vi "add address to register list.vi"(0 "reference":refnum<vi>, 7 "RegisterAddress":i32, 13 "Register Selected":bool) -> ()   [LabVIEW 2010]
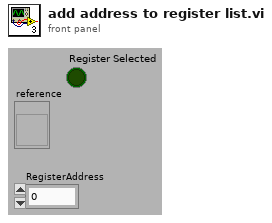
[diagram p1: front panel]
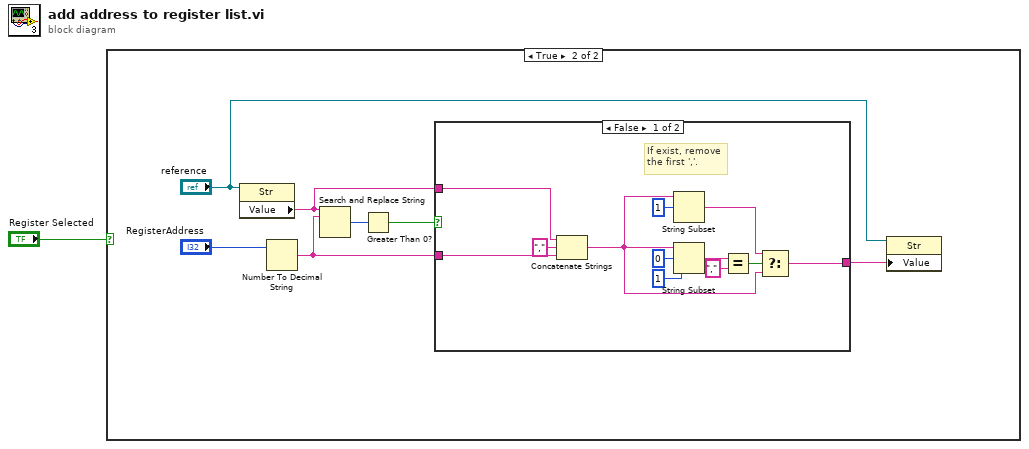
[diagram p0: block diagram]
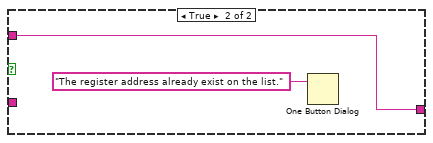
[diagram p3: hidden frame]
diagram:
  n1 = case shown="True" "Register Selected" {
    frame False {
    }
    frame True {
      n2 = property class="Str"(reference="reference") -> ("Value"=w8:string)  [unwired: 1 in, 2 out]
      n3 = Number To Decimal String(number="RegisterAddress") -> (decimal integer string=w6:string)  [unwired: 1 in]
      n4 = Search and Replace String(input string=w8, search string=w6) -> (number of replacements=w5:i32)  [unwired: 6 in, 3 out]
      n5 = Greater Than 0?(x=w5) -> (x > 0?=w7:bool)
      n6 = case shown="False" w7 {
        tunnel: w6 -> [w11 _]
        tunnel: w8 -> [w10 w21]
        tunnel: [w9 w21] -> w3
        frame False {
          # "If exist, remove\nthe first ','."
          n7 = Concatenate Strings(w10, "," ("string"), w11) -> (w12:string)
          n8 = String Subset(string=w12, offset (0)=1) -> (substring=w13:string)  [unwired: 1 in]
          n9 = String Subset(string=w12, offset (0)=0, length (rest)=1 ("length (rest)")) -> (substring=w17:string)
          n10 = Equal?(x=w17, y=",") -> (x = y?=w15:bool)
          n11 = Select(t=w13, s=w15, f=w12) -> (s? t:f=w9:string)
        }
        frame True {
          n12 = One Button Dialog(message="The register address already exist on the list.") -> ()  [unwired: 1 in, 1 out]
        }
      }
      n13 = property class="Str"(reference="reference", "Value"=w3) -> ()  [unwired: 1 in, 2 out]
    }
  }
